vi "Find Goal Angle Difference.vi"(6 "Goal Display 2":T1(plugin-control), 10 "Normalized Rect":T2, 11 "Camera Type":T3) -> (3 "Angle Diff":dbl)   [LabVIEW 2015]
uses:
  Camera Types.ctl
panel:
  out "x*y":dbl
  out "Angle Difference":dbl
  out "View Distance":dbl
  out "Right Distance":dbl
  out "Left Distance":dbl
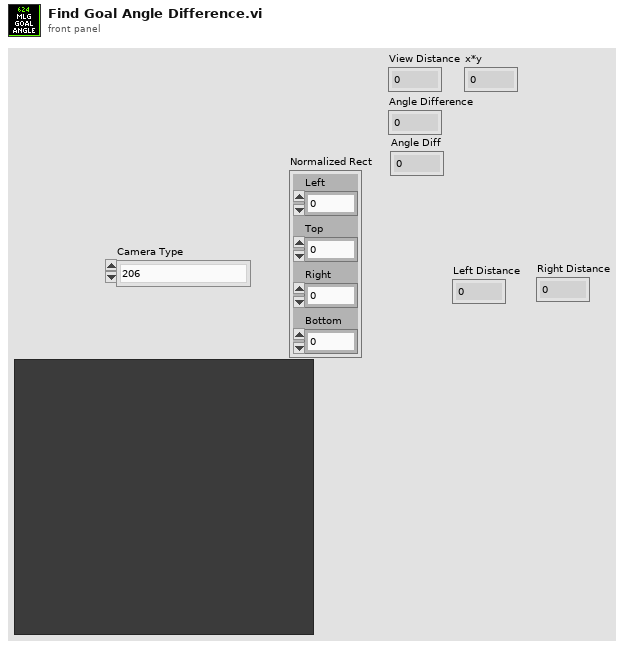
[diagram p1: front panel]
types:
  T1 = typedef "IMAQ Image.ctl" = refnum<image>
  T2 = cluster{"Left":dbl, "Top":dbl, "Right":dbl, "Bottom":dbl}
  T3 = typedef "Camera Types.ctl" = enum16{"206", "1011", "1013", "MS HD3000 square", "MS HD3000 640x480"}
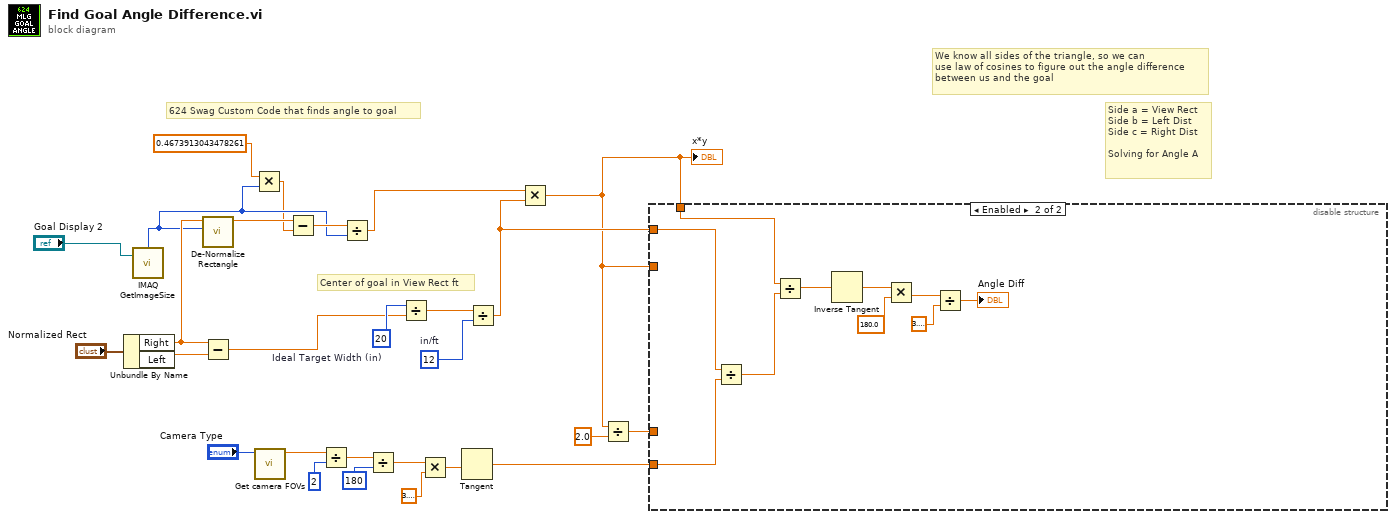
[diagram p0: block diagram]
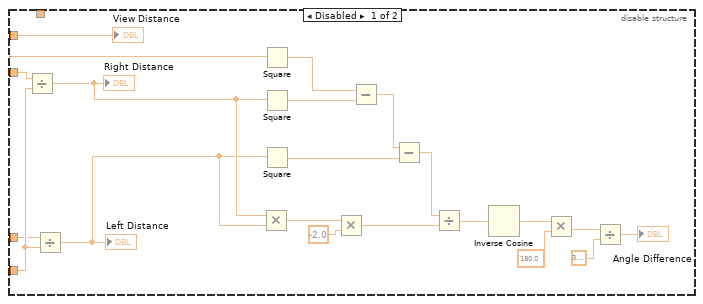
[diagram p2: hidden frame]
diagram:
  w17 = 20  # Ideal Target Width (in)
  w21 = 12  # in/ft
  # "Side a = View Rect\nSide b = Left Dist\nSide c = Right Dist\n\nSolving for Angle A"
  # "We know all sides of the triangle, so we can\nuse law of cosines to figure out the angle difference\nbetween us and the goal"
  # "Center of goal in View Rect ft"
  # "624 Swag Custom Code that finds angle to goal"
  n1 = Unbundle By Name("Normalized Rect") -> ("Right"=w12:dbl, "Left"=w11:dbl)
  n2 = call "IMAQ GetImageSize"("Image"="Goal Display 2") -> ("X Resolution"=w4:i32)  [unwired: 3 in, 2 out]
  n3 = call "De-Normalize Rectangle.vi"("X Resolution"=w4, "Right"=w12) -> ("Pixels"=w10:dbl)  [unwired: 9 in]
  n4 = Subtract(x=w12, y=w11) -> (x-y=w14:dbl)
  n5 = Multiply(x=0.4673913043478261, y=w4) -> (x*y=w2:dbl)
  n6 = call "Get camera FOVs.vi"("Camera Type"="Camera Type") -> ("FOV"=w19:dbl)  [unwired: 9 in, 1 out]
  n7 = Subtract(x=w10, y=w2) -> (x-y=w9:dbl)
  n8 = Divide(x=w19, y=2) -> (x/y=w25:dbl)
  n9 = Divide(x=w9, y=w4) -> (x/y=w8:dbl)
  n10 = Divide(x=w25, y=180) -> (x/y=w24:dbl)
  n11 = Divide(x=w17, y=w14) -> (x/y=w20:dbl)
  n12 = Multiply(x=w24, y=3.141592653589793) -> (x*y=w26:dbl)
  n13 = Tangent(1:w26) -> (0:w16:dbl)
  n14 = Divide(x=w20, y=w21) -> (x/y=w7:dbl)
  n15 = Multiply(x=w8, y=w7) -> (x*y=w1:dbl)
  "x*y" <- w1
  n16 = Divide(x=w1, y=2.0) -> (x/y=w5:dbl)
  n17 = disable-structure shown="Enabled" {
    disable-tunnel: w16 -> [w47 w57]
    disable-tunnel: w7 -> [w30 w56]
    disable-tunnel: w5 -> [w29 _]
    disable-tunnel: w1 -> [w28 _]
    disable-tunnel: w1 -> [_ w55]
    frame Disabled {
      n18 = Divide(x=w28, y=w47) -> (x/y=w42:dbl)
      "Right Distance" <- w42
      n19 = Divide(x=w29, y=w47) -> (x/y=w41:dbl)
      "Left Distance" <- w41
      n20 = Multiply(x=w42, y=w41) -> (x*y=w40:dbl)
      n21 = Square(x=w30) -> (x^2=w46:dbl)
      n22 = Square(x=w42) -> (x^2=w45:dbl)
      n23 = Square(x=w41) -> (x^2=w43:dbl)
      n24 = Multiply(x=w40, y=-2.0) -> (x*y=w37:dbl)
      n25 = Subtract(x=w46, y=w45) -> (x-y=w44:dbl)
      n26 = Subtract(x=w44, y=w43) -> (x-y=w38:dbl)
      n27 = Divide(x=w38, y=w37) -> (x/y=w36:dbl)
      n28 = Inverse Cosine(1:w36) -> (0:w35:dbl)
      n29 = Multiply(x=w35, y=180.0) -> (x*y=w33:dbl)
      n30 = Divide(x=w33, y=3.141592653589793) -> (x/y=→"Angle Difference":dbl)
      "View Distance" <- w30
    }
    frame Enabled {
      n31 = Divide(x=w56, y=w57) -> (x/y=w54:dbl)
      n32 = Divide(x=w55, y=w54) -> (x/y=w53:dbl)
      n33 = Inverse Tangent(1:w53) -> (0:w49:dbl)
      n34 = Multiply(x=w49, y=180.0) -> (x*y=w51:dbl)
      n35 = Divide(x=w51, y=3.141592653589793) -> (x/y=→"Angle Diff":dbl)
    }
  }
